vi "Set configuration chain.vi"(8 "error in (no error)":errorcluster, 9 "class names":string[](array[string]), 10 "configuration":variant[](array[variant]), 11 "StageSPIM in":refnum<class "StageSPIM.lvclass">) -> (0 "error out":errorcluster, 3 "StageSPIM out":refnum<class "StageSPIM.lvclass">)   [LabVIEW 2012, in "StageSPIM.lvclass"]
uses:
  StageSPIM.lvclass
  <vilib>/Distrio/Murmex/Murmex/Murmex.lvclass
  StageSPIM.lvclass/StageSPIM.ctl
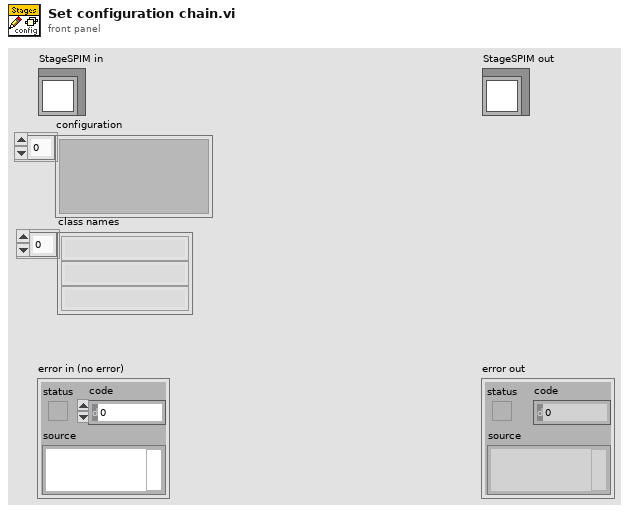
[diagram p1: front panel]
types:
  T1 = typedef "StageSPIM.lvclass/configuration_cluster.ctl" = cluster{"Port":T2, "Baudrate":T3, "Update frequency":dbl[unit], "S/N Master controller":string, "Interface":T4, "soft min limit":dbl[], "soft max limit":dbl[], "startup speedA":dbl[unit], "startup speedX":dbl[unit], "startup speedY":dbl[unit], "startup speedZ":dbl[unit]}
  T2 = typedef "StageSPIM.lvclass/port_control.ctl" = i32
  T3 = typedef "StageSPIM.lvclass/baud_rate_control.ctl" = u16
  T4 = typedef "StageSPIM.lvclass/connection_type.ctl" = enum16{"RS232", "RS232 DaisyChain", "USB", "USB_DaisyChain"}
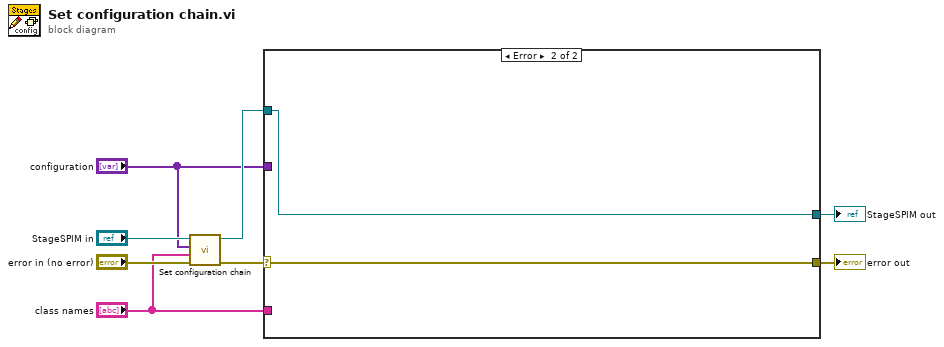
[diagram p0: block diagram]
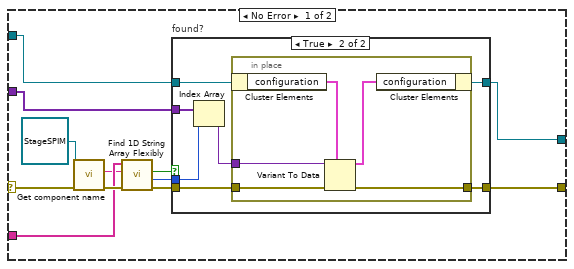
[diagram p2: hidden frame]
diagram:
  n1 = call-parent "Set configuration chain.vi"("error in (no error)"="error in (no error)", "class names"="class names", "configuration"="configuration", "Murmex in"="StageSPIM in") -> ("error out"=w6:errorcluster, "Murmex out"=w5:refnum<class "StageSPIM.lvclass">)  [unwired: 6 in]
  n2 = case shown="Error" w6 {
    selector: w6 -> [w20 w35]
    tunnel: w5 -> [w13 w36]
    tunnel: "configuration" -> [w14 _]
    tunnel: "class names" -> [w17 _]
    tunnel: [w10 w36] -> w2
    tunnel: [w9 w35] -> w1
    frame No Error {
      n3 = call <vilib>:"Get component name.vi"("error in (no error)"=w20, "Murmex in"=refnum<class "StageSPIM.lvclass"> refnum ("StageSPIM.lvclass")) -> ("error out"=w18:errorcluster, "component name"=w16:string)  [unwired: 7 in, 1 out]
      n4 = call <vilib>:"Find 1D String Array Flexibly.vi"("error in (no error)"=w18, "element"=w16, "array"=w17) -> ("error out"=w15:errorcluster, "index of element"=w12:i32, "found?"=w11:bool)  [unwired: 6 in]
      n5 = case "found?" shown="True" w11 {
        tunnel: w12 -> [_ w28]
        tunnel: w15 -> [w22 w27]
        tunnel: [w22 w26] -> w9
        tunnel: [w21 w24] -> w10
        tunnel: w14 -> [_ w29]
        tunnel: w13 -> [w21 w23]
        frame False {
        }
        frame True {
          n6 = Index Array(array=w29, index=w28) -> (element=w25:variant)
          n7 = in-place {
            in-place-border: w27 -> [w34]
            in-place-border: [w33] -> w26
            in-place-border: w25 -> [w30]
            n8 = in-place-cluster #1(w23) -> ("configuration"=w32:T1)
            n9 = Variant To Data(error in=w34, type=w32, Variant=w30) -> (data=w31:T1, error out=w33:errorcluster)
            n10 = in-place-cluster #1("configuration"=w31) -> (w24:refnum<class "StageSPIM.lvclass">)
          }
        }
      }
    }
    frame Error {
    }
  }
  "error out" <- w1
  "StageSPIM out" <- w2
